vi "Time-Delayed Send Message.vi"(6 "Message Priority (Normal)":T1=enum."Normal", 7 "# Copies (0 = infinite repeat)":u32, 8 "error in (no error)":errorcluster, 9 "Milliseconds To Wait":i32=1000, 10 "Message":refnum<class "Message.lvclass">, 11 "Message Enqueuer":refnum<class "Message Enqueuer.lvclass">) -> (0 "error out":errorcluster, 2 "Delivery Notifier":refnum<notifier>)   [LabVIEW 2019, in "AF_Messages-PPL.lvlib"]
doc: "Waits for the specified amount of time and then sends a message to an actor a specified number of times."
uses:
  AF_Messages-PPL.lvlib
  PPLs/Actor Framework.lvlibp/Message Enqueuer/Message Enqueuer.lvclass
  PPLs/Actor Framework.lvlibp/Message/Message.lvclass
  Time-Delay Override Options.ctl
  PPLs/Actor Framework.lvlibp/Message Enqueuer/Message Priority.ctl
  Time-Delayed Send Message Core.vi
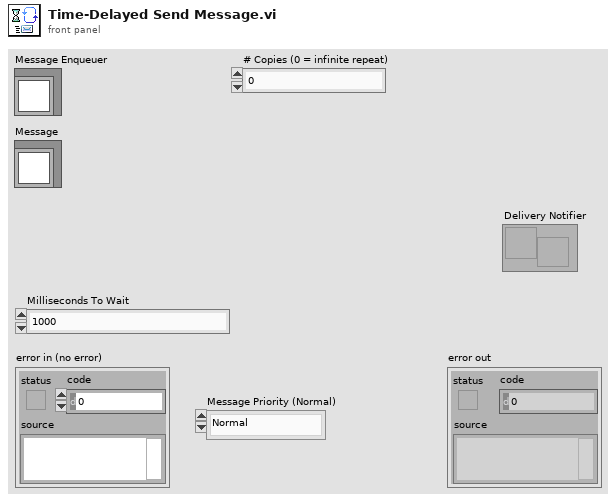
[diagram p1: front panel]
types:
  T1 = typedef "Actor Framework.lvlibp/Message Enqueuer.lvclass/Message Priority.ctl" = enum16{"Low", "Normal", "High"}
  T2 = typedef "AF_Messages-PPL.lvlib/Time-Delay Override Options.ctl" = enum16{"Send next copy now", "Skip next scheduled copy", "Send next copy now and stop all further copies", "Stop all further copies"}
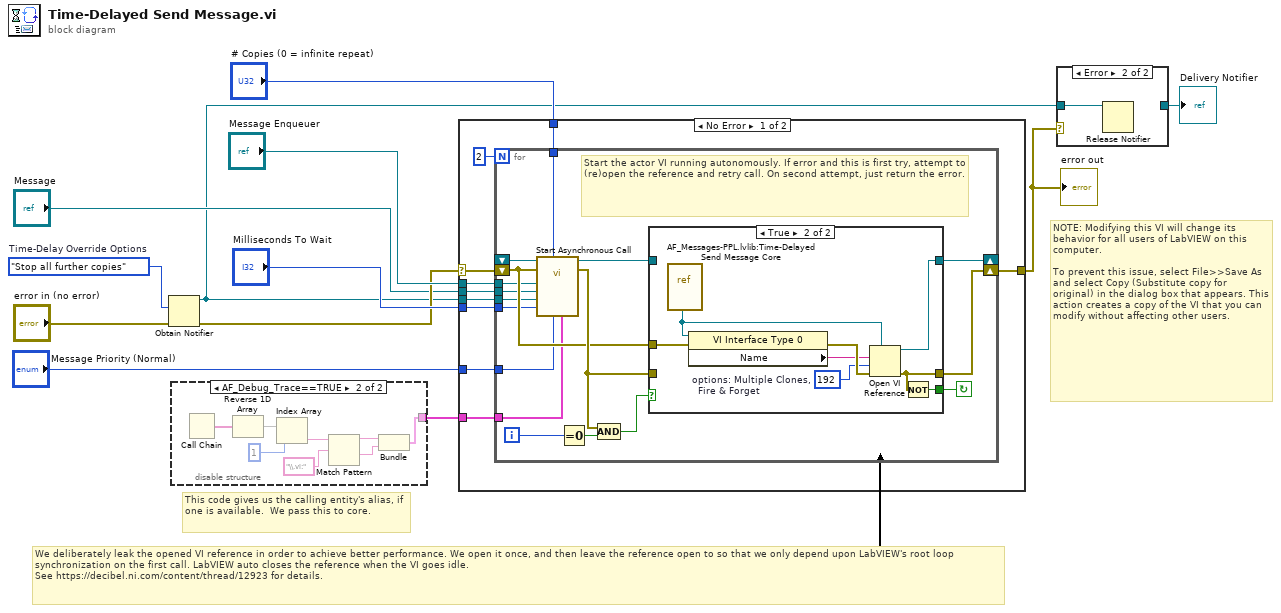
[diagram p0: block diagram]
diagram:
  w12 = Time-Delay_Override_Options."Stop all further copies"  # Time-Delay Override Options
  # "This code gives us the calling entity's alias, if one is available.  We pass this to core."
  # "We deliberately leak the opened VI reference in order to achieve better performance. We open it once, and then leave the reference open to so that we only depend upon LabVIEW's root loop synchronization on the first call. LabVIEW auto closes the reference when the VI goes idle. \nSee https://decibel.ni.com/content/thread/12923 for details."
  # "NOTE: Modifying this VI will change its behavior for all users of LabVIEW on this computer.\n\nTo prevent this issue, select File>>Save As and select Copy (Substitute copy for original) in the dialog box that appears. This action creates a copy of the VI that you can modify without affecting other users."
  n1 = Obtain Notifier(notification data type=w12, error in (no error)="error in (no error)") -> (notifier out=w2:refnum<notifier>, error out=w4:errorcluster)  [unwired: 2 in, 1 out]
  n2 = disable-structure shown="AF_Debug_Trace==TRUE" {
    disable-tunnel: [_ w18] -> w1
    frame condition #0 (active) {
    }
    frame condition #1 {
      n3 = Call Chain() -> (call chain=w17:string[])
      n4 = Reverse 1D Array(array=w17) -> (reversed array=w16:string[])
      n5 = Index Array(array=w16, index=1) -> (element=w15:string)
      n6 = Match Pattern(string=w15, regular expression="\\.vi:") -> (before substring=w20:string, after substring=w19:string)  [unwired: 1 in, 2 out]
      n7 = Bundle(w20, w19) -> (w18:cluster{string, string})  [unwired: 1 in]
    }
  }
  n8 = case shown="No Error" w4 {
    selector: w4 -> [w28 w58]
    tunnel: [w29 w58] -> w5
    tunnel: "Message Priority (Normal)" -> [w27 _]
    tunnel: "Milliseconds To Wait" -> [w26 _]
    tunnel: "Message" -> [w25 _]
    tunnel: w2 -> [w24 _]
    tunnel: "Message Enqueuer" -> [w23 _]
    tunnel: "# Copies (0 = infinite repeat)" -> [w22 _]
    tunnel: w1 -> [w21 _]
    frame No Error {
      n9 = for {
        N: 2 -> [_]
        shift-right: [w47] -> _
        shift-left: _ -> [w39]
        shift-right: [w46] -> w29
        shift-left: w28 -> [w40]
        tunnel: w27 -> [w37]
        tunnel: w26 -> [w36]
        tunnel: w25 -> [w35]
        tunnel: w24 -> [w34]
        tunnel: w23 -> [w33]
        tunnel: w22 -> [w32]
        tunnel: w21 -> [w31]
        i -> [w43]
        stop <- w41 continue-if-true
        # "Start the actor VI running autonomously. If error and this is first try, attempt to (re)open the reference and retry call. On second attempt, just return the error."
        n10 = call-by-ref "Start Asynchronous Call"(reference=w39, error in=w40, "Caller Info"=w31, "Message Priority (Normal)"=w37, "How Many Copies (0 = infinite repeat)"=w32, "Time To Wait"=w36, "Delivery Notifier"=w34, "Message"=w35, "Message Enqueuer"=w33) -> (reference out=w38:refnum<vi>, error out=w42:errorcluster)  [unwired: 5 in]
        n11 = Equal To 0?(x=w43) -> (x = 0?=w44:bool)
        n12 = Compound Arithmetic op=AND(w42, w44) -> (w45:bool)
        n13 = case shown="True" w45 {
          tunnel: [w49 w54] -> w47
          tunnel: [w48 w52] -> w46
          tunnel: w38 -> [w49 _]
          tunnel: w42 -> [w48 _]
          tunnel: [_ w53] -> w41
          tunnel: w40 -> [_ w51]
          frame False {
          }
          frame True {
            w55 = 192  # options: Multiple Clones,   Fire & Forget
            n14 = vi-ref "AF_Messages-PPL.lvlib:Time-Delayed Send Message Core.vi"() -> (w50:refnum<vi>)
            n15 = property class="VI Interface Type 0"(reference=w50, error in=w51) -> (error out=w57:errorcluster, "Name"=w56:string)  [unwired: 1 out]
            n16 = Open VI Reference(type specifier VI Refnum (for type only)=w50, vi path=w56, options=w55, error in (no error)=w57) -> (vi reference=w54:refnum<vi>, error out=w52:errorcluster)  [unwired: 2 in]
            n17 = Not(x=w52) -> (.not. x?=w53:bool)
          }
        }
      }
    }
    frame Error {
    }
  }
  "error out" <- w5
  n18 = case shown="Error" w5 {
    tunnel: [w59 _] -> w10
    tunnel: w2 -> [w59 w60]
    frame No Error {
    }
    frame Error {
      n19 = Release Notifier(notifier=w60) -> ()  [unwired: 2 in, 3 out]
    }
  }
  "Delivery Notifier" <- w10
